vi "theOne_V2.vi"() -> ()   [LabVIEW 2021]
uses:
  <userlib>/er4commlib_labview/er4commlib_labview.lvlib
panel:
  in  "acqFlag":bool
  in  "purgeFlag":bool
  out "DataCh1":dbl[](graph)
  out "DataCh2":dbl[](graph)
  out "DataCh3":dbl[](graph)
  out "DataCh4":dbl[](graph)
  out "VolAndTrig":dbl[][](graph)
  out "triggerImage":picture
  in  "path to triggerImage file jpg":path=path "C:/neoDiag/MrAnderson/Img/trigger.jpg"
  in  "Trigger":T1={"manual start"=FALSE, "duration [us]"=200.0, "period [ms]"=1.0, "delay [us]"=0.0, "reps"=1000, "active"=TRUE} {"delay [us]" format="%_5f"; "period [ms]" format="%_5f"; "duration [us]" format="%_5f"}
  in  "Voltage Stimulus":T2={"stimulus"=FALSE, "Vhold [mV]"=-50.0, "Vpulse [mV]"=0.0, "Vstep [mV]"=10.0, "N"=10, "Thold [ms]"=0.0, "Tpulse [ms]"=200.0} {"Tpulse [ms]" format="%_5f"; "Thold [ms]" format="%_5f"; "Vstep [mV]" format="%_5f"; "Vpulse [mV]" format="%_5f"; "Vhold [mV]" format="%_5f"}
  in  "acquire data":bool
  in  "stop":bool
  out "pulseTrainImage":picture
  in  "path to pulseTrainImage file jpg":path=path "C:/neoDiag/MrAnderson/Img/volProtVarAmpl.jpg"
  in  "Tab Control":enum32{"AcqPara", "AdvPara"}(tab)
  in  "Acquisition Parameters":T3={"Camera "=FALSE, "Period [ms]"=200.0, "Duration [ms]"=0.2, "Delay [ms]"=0.0, "Pulses [#]"=10, "sampling rate [kHz]"="1,25", "current range [nA]"="2", "time [s]"=2.0} {"Delay [ms]" format="%_5f"; "Duration [ms]" format="%_5f"; "Period [ms]" format="%_5f"}
  in  "advancedSettings":T4={"Channels to read"=6, "update rate of read data loop"=100, "displayRange"=512}
  out "Error Out Int":u32
  out "Error Out String":string="clean"
  out "E4 parameters":T5={"currentChannelsNum out"=1, "voltageChannelsNum out"=4, "gpChannelsNum out"=1, "sampling rate [kHz]"=1.25, "real sampling rate [kHz]"=1.220703125, "Ch_min"=-2.0, "Ch_max"=2.0, "Ch_step"=6.103701895199438e-05, "Ch_unit"=1e-09}
  in  "Display 1":cluster{"ChArray":bool[]}={"ChArray"=[FALSE, TRUE, TRUE, TRUE, FALSE, FALSE]}
  out "Error Read":errorcluster
  # "DataCh1"
  # "DataCh2"
  # "DataCh3"
  # "DataCh4"
  # "Voltage"
  # "Trigger"
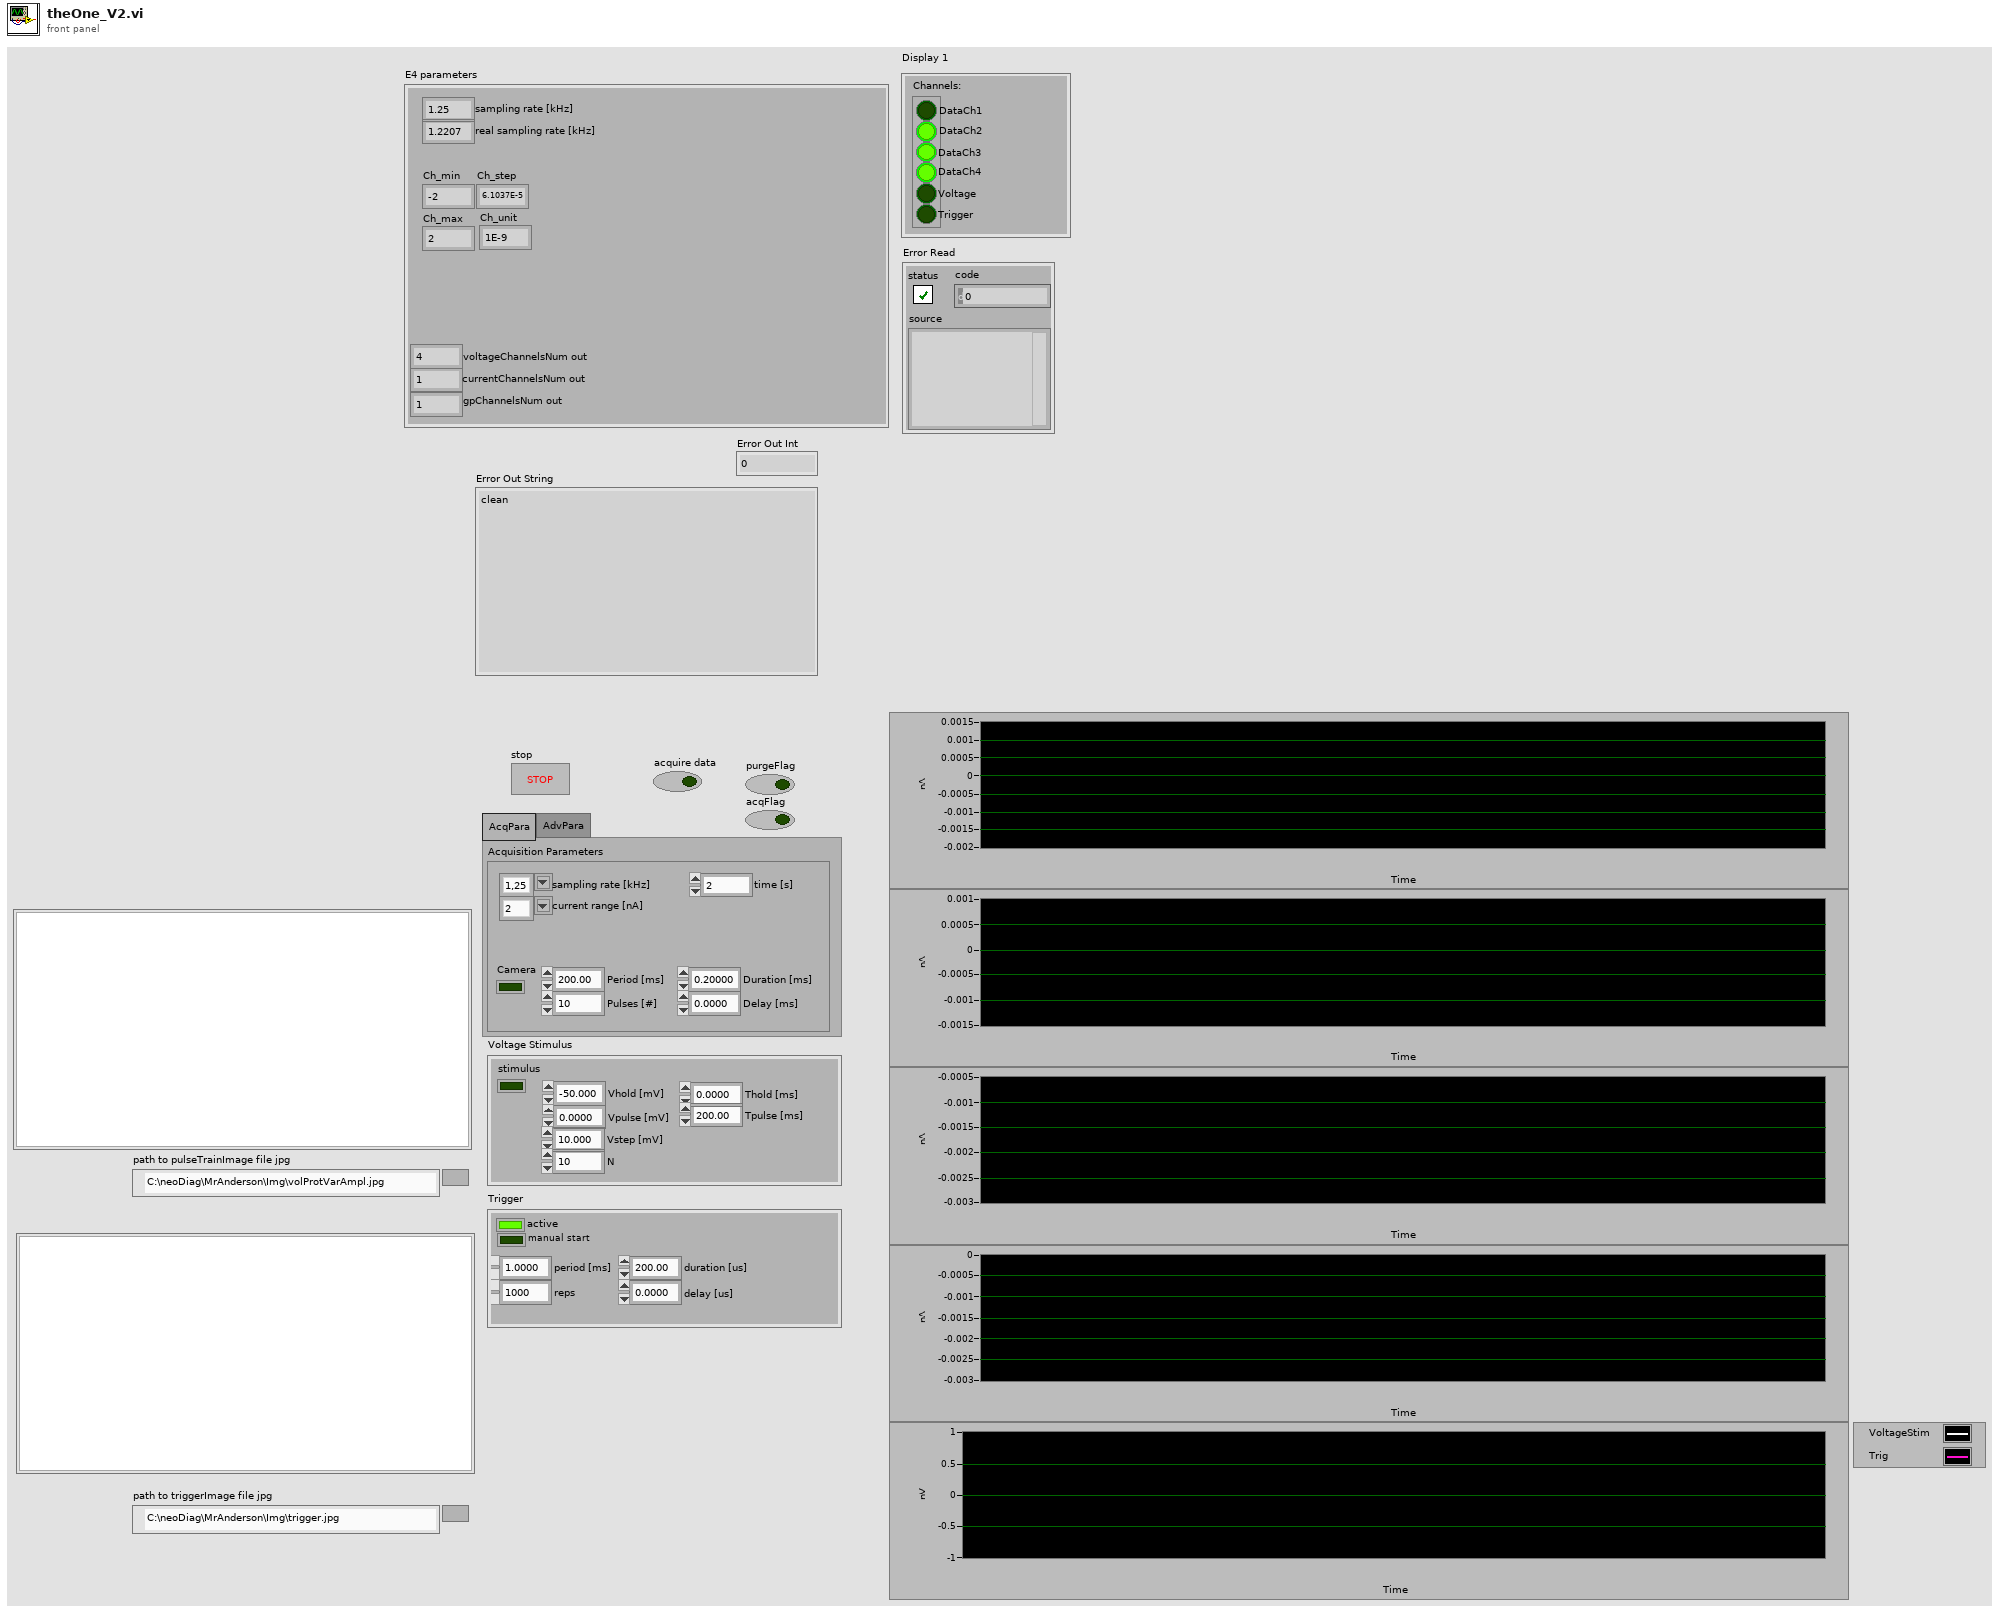
[diagram p1: front panel]
types:
  T1 = cluster{"manual start":bool, "duration [us]":dbl, "period [ms]":dbl, "delay [us]":dbl, "reps":u32, "active":bool}
  T2 = cluster{"stimulus":bool, "Vhold [mV]":dbl, "Vpulse [mV]":dbl, "Vstep [mV]":dbl, "N":u32, "Thold [ms]":dbl, "Tpulse [ms]":dbl}
  T3 = cluster{"Camera ":bool, "Period [ms]":dbl, "Duration [ms]":dbl, "Delay [ms]":dbl, "Pulses [#]":u32, "sampling rate [kHz]":string, "current range [nA]":string, "time [s]":dbl}
  T4 = cluster{"Channels to read":i32, "update rate of read data loop":i32, "displayRange":i32}
  T5 = cluster{"currentChannelsNum out":u32, "voltageChannelsNum out":u32, "gpChannelsNum out":u32, "sampling rate [kHz]":dbl, "real sampling rate [kHz]":dbl, "Ch_min":dbl, "Ch_max":dbl, "Ch_step":dbl, "Ch_unit":dbl}
  T6 = typedef "imagedata.ctl" = cluster{"image type":i32, "image depth":i32, "image":u8[], "mask":u8[], "colors":u32[], "Rectangle":cluster{"left":i16, "top":i16, "right":i16, "bottom":i16}}
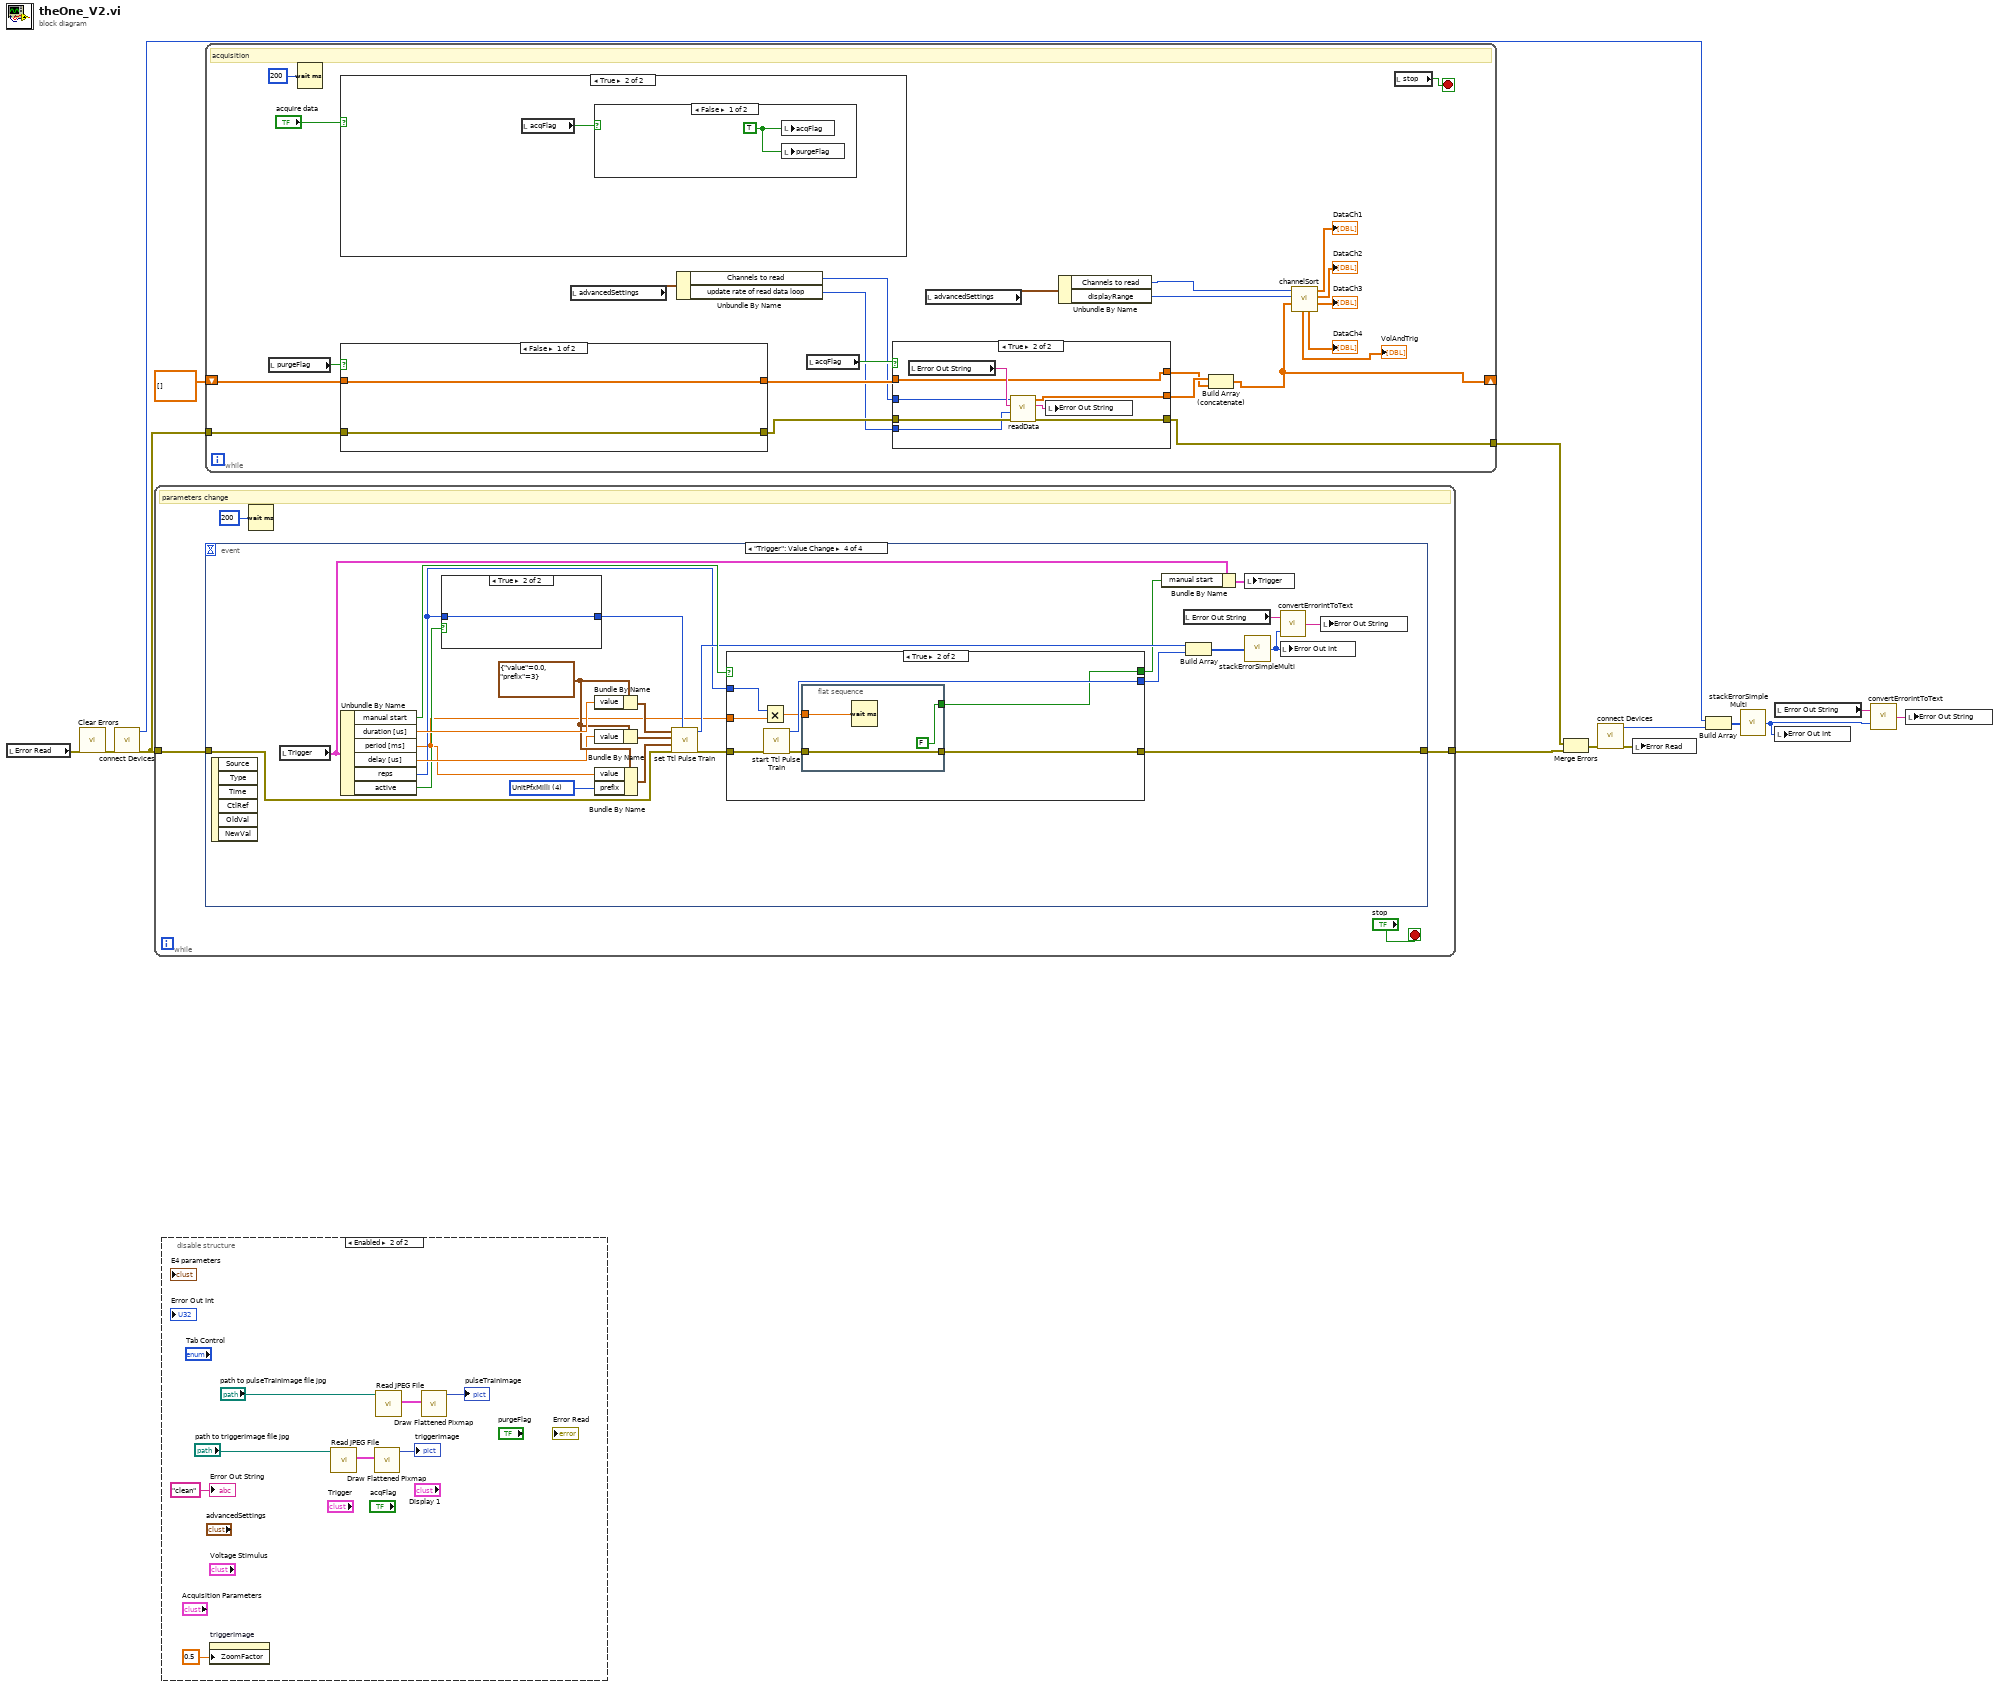
[diagram p0: block diagram]
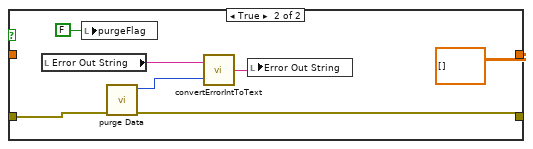
[diagram p2: hidden frame]
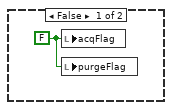
[diagram p3: hidden frame]
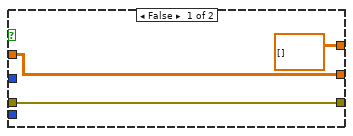
[diagram p5: hidden frame]
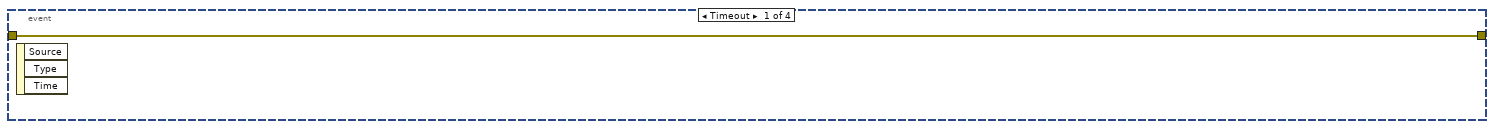
[diagram p6: hidden frame]
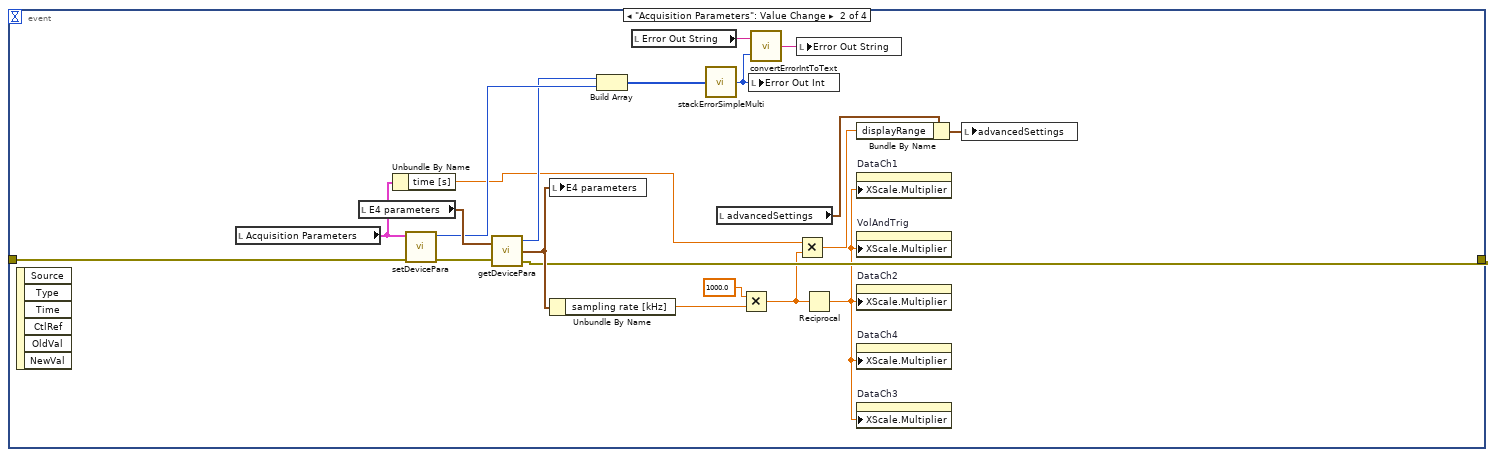
[diagram p7: hidden frame]
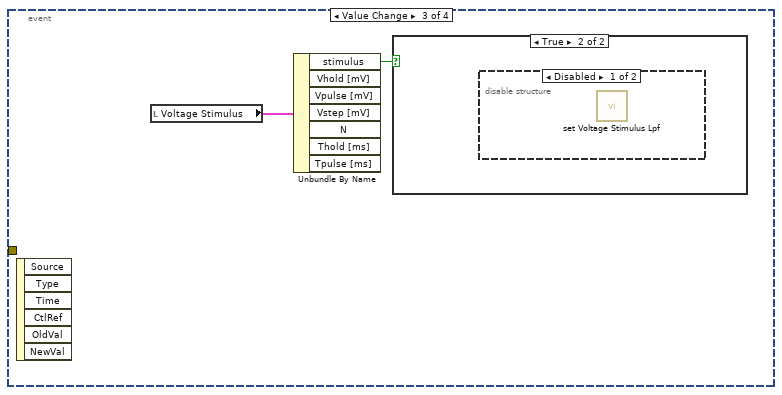
[diagram p8: hidden frame]
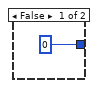
[diagram p11: hidden frame]
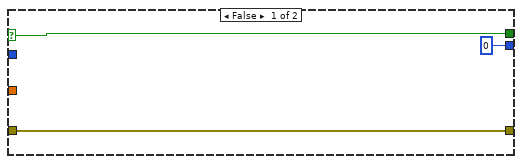
[diagram p12: hidden frame]
diagram:
  n1 = local read "Error Read"() -> (w13:errorcluster)
  n2 = call <vilib>:"Clear Errors.vi"("error in (no error)"=w13) -> ("error out"=w11:errorcluster)  [unwired: 5 in, 1 out]
  n3 = call <userlib>:"connect Devices.vi"("error in (no error)"=w11) -> ("error out"=w2:errorcluster, "function return"=w3:u32)  [unwired: 9 in]
  n4 = while {
    tunnel: w2 -> [w16]
    tunnel: [w15] -> w1
    stop <- "stop" stop-if-true
    # "parameters change"
    n5 = event shown="[3] \"Trigger\": Value Change" {
      selector: _ -> [_ _ _ _]
      dyn-events: _ -> [_ _ _ _]
      timeout: _ -> [_ _ _ _]
      tunnel: [w19 w32 _ w64] -> w15
      tunnel: w16 -> [w19 w31 _ w56]
      event Timeout {
        n6 = event-data() -> ()  [unwired: 1 in, 3 out]
      }
      event "Acquisition Parameters": Value Change {
        n7 = event-data() -> ()  [unwired: 1 in, 6 out]
        n8 = local read "Acquisition Parameters"() -> (w25:T3)
        n9 = local read "E4 parameters"() -> (w34:T5)
        n10 = Unbundle By Name(w25) -> ("time [s]"=w24:dbl)
        n11 = call "setDevicePara.vi"("error in (no error)"=w31, "Acquisition Parameters 2"=w25) -> ("error out"=w38:errorcluster, "function return"=w30:u32)  [unwired: 8 in]
        n12 = call "getDevicePara.vi"("Seetings in"=w34, "error in (no error)"=w38) -> ("Error Out"=w29:u32, "Seetings out"=w37:T5, "error out"=w32:errorcluster)
        n13 = local write "E4 parameters"(w37) -> ()
        n14 = Unbundle By Name(w37) -> ("sampling rate [kHz]"=w39:dbl)
        n15 = Build Array(w29, w30) -> (w28:u32[])
        n16 = local read "Error Out String"() -> (w36:string)
        n17 = call "stackErrorSimpleMulti.vi"("Error List"=w28) -> ("Error Out"=w27:u32)
        n18 = local read "advancedSettings"() -> (w20:T4)
        n19 = Multiply(x=1000.0, y=w39) -> (x*y=w23:dbl)
        n20 = local write "Error Out Int"(w27) -> ()
        n21 = call "convertErrorIntToText.vi"("Error Int In (function return)"=w27, "Error String In"=w36) -> ("Error String Out"=w35:string)
        n22 = local write "Error Out String"(w35) -> ()
        n23 = Multiply(x=w24, y=w23) -> (x*y=w21:dbl)
        n24 = Reciprocal(x=w23) -> (1/x=w26:dbl)
        n25 = Bundle By Name(cluster=w20, "displayRange"=w21) -> (w22:T4)
        n26 = property on="DataCh1" class="WFGraph (strict)"("XScale.Multiplier"=w26) -> ()  [unwired: 2 in, 2 out]
        n27 = property on="VolAndTrig" class="WFGraph (strict)"("XScale.Multiplier"=w26) -> ()  [unwired: 2 in, 2 out]
        n28 = property on="DataCh2" class="WFGraph (strict)"("XScale.Multiplier"=w26) -> ()  [unwired: 2 in, 2 out]
        n29 = property on="DataCh4" class="WFGraph (strict)"("XScale.Multiplier"=w26) -> ()  [unwired: 2 in, 2 out]
        n30 = property on="DataCh3" class="WFGraph (strict)"("XScale.Multiplier"=w26) -> ()  [unwired: 2 in, 2 out]
        n31 = local write "advancedSettings"(w22) -> ()
      }
      event "Voltage Stimulus.stimulus": Value Change {
        n32 = event-data() -> ()  [unwired: 1 in, 6 out]
        n33 = local read "Voltage Stimulus"() -> (w41:T2)
        n34 = Unbundle By Name(w41) -> ("stimulus"=w40:bool)  [unwired: 6 out]
        n35 = case shown="True" w40 {
          frame False {
          }
          frame True {
            n36 = disable-structure shown="Disabled" {
              frame Disabled {
                n37 = call <userlib>:"set Voltage Stimulus Lpf.vi"() -> ()  [unwired: 10 in, 2 out]
              }
              frame Enabled {
              }
            }
          }
        }
      }
      event "Trigger": Value Change {
        w59 = cluster{"value":dbl, "prefix":u32} {"value"=0.0, "prefix"=3} ("pulseDuration")
        w63 = u32 4 items=["UnitPfxFemto", "UnitPfxPico", "UnitPfxNano", "UnitPfxMicro", "UnitPfxMilli", "UnitPfxNone", "UnitPfxKilo", "UnitPfxMega", "UnitPfxGiga", "UnitPfxTera", "UnitPfxPeta", "UnitPfxNum"] ("prefix")
        n38 = event-data() -> ()  [unwired: 1 in, 6 out]
        n39 = local read "Trigger"() -> (w46:T1)
        n40 = Unbundle By Name(w46) -> ("manual start"=w65:bool, "duration [us]"=w61:dbl, "period [ms]"=w42:dbl, "delay [us]"=w58:dbl, "reps"=w43:u32, "active"=w54:bool)
        n41 = case shown="True" w54 {
          tunnel: w43 -> [_ w67]
          tunnel: [u32 0 ("reps") w67] -> w53
          frame False {
          }
          frame True {
          }
        }
        n42 = Bundle By Name(cluster=w59, "value"=w61) -> (w60:cluster{"value":dbl, "prefix":u32})
        n43 = Bundle By Name(cluster=w59, "value"=w58) -> (w57:cluster{"value":dbl, "prefix":u32})
        n44 = Bundle By Name(cluster=w59, "value"=w42, "prefix"=w63) -> (w62:cluster{"value":dbl, "prefix":u32})
        n45 = call <userlib>:"set Ttl Pulse Train.vi"("numberOfPulses"=w53, "error in (no error)"=w56, "period"=w62, "pulseDelay"=w57, "pulseDuration"=w60) -> ("error out"=w55:errorcluster, "function return"=w49:u32)  [unwired: 5 in]
        n46 = case shown="True" w65 {
          selector: w65 -> [w68 _]
          tunnel: w55 -> [w70 w78]
          tunnel: [w70 w74] -> w64
          tunnel: [u32 0 ("function return") w77] -> w48
          tunnel: [w68 w76] -> w45
          tunnel: w43 -> [_ w73]
          tunnel: w42 -> [_ w72]
          frame False {
          }
          frame True {
            n47 = Multiply(x=w73, y=w72) -> (x*y=w71:dbl)
            n48 = call <userlib>:"start Ttl Pulse Train.vi"("error in (no error)"=w78) -> ("error out"=w75:errorcluster, "function return"=w77:u32)  [unwired: 9 in]
            n49 = flat-sequence {
              tunnel: [FALSE] -> w76
              tunnel: w75 -> [w80]
              tunnel: [w80] -> w74
              tunnel: w71 -> [w79]
              frame #0 {
                n50 = Wait (ms)(milliseconds to wait=w79) -> ()  [unwired: 1 out]
              }
            }
          }
        }
        n51 = Bundle By Name(cluster=w46, "manual start"=w45) -> (w44:T1)
        n52 = local read "Error Out String"() -> (w47:string)
        n53 = Build Array(w49, w48) -> (w51:u32[])
        n54 = local write "Trigger"(w44) -> ()
        n55 = call "stackErrorSimpleMulti.vi"("Error List"=w51) -> ("Error Out"=w50:u32)
        n56 = call "convertErrorIntToText.vi"("Error Int In (function return)"=w50, "Error String In"=w47) -> ("Error String Out"=w52:string)
        n57 = local write "Error Out Int"(w50) -> ()
        n58 = local write "Error Out String"(w52) -> ()
      }
    }
    n59 = Wait (ms)(milliseconds to wait=u32 200) -> ()  [unwired: 1 out]
  }
  n60 = disable-structure shown="Enabled" {
    frame Disabled {
    }
    frame Enabled {
      n61 = property on="triggerImage" class="Pict"("ZoomFactor"=sgl 0.5 ("Zoom Factor")) -> ()  [unwired: 2 in, 2 out]
      n62 = call <vilib>:"Read JPEG File.vi"("path to JPEG file"="path to triggerImage file jpg") -> ("image data"=w85:T6)  [unwired: 8 in, 2 out]
      n63 = call <vilib>:"Draw Flattened Pixmap.vi"("image data"=w85) -> ("new picture"=→"triggerImage":picture)  [unwired: 8 in]
      n64 = call <vilib>:"Read JPEG File.vi"("path to JPEG file"="path to pulseTrainImage file jpg") -> ("image data"=w88:T6)  [unwired: 8 in, 2 out]
      n65 = call <vilib>:"Draw Flattened Pixmap.vi"("image data"=w88) -> ("new picture"=→"pulseTrainImage":picture)  [unwired: 8 in]
      "Error Out String" <- "clean" ("Error String Out")
    }
  }
  n66 = while {
    tunnel: w2 -> [w106]
    shift-right: [w90] -> _
    shift-left: dbl[][] [] -> [w105]
    tunnel: [w102] -> w12
    stop <- w110 stop-if-true
    # "acquisition"
    n67 = local read "purgeFlag"() -> (w108:bool)
    n68 = Wait (ms)(milliseconds to wait=u32 200) -> ()  [unwired: 1 out]
    n69 = case shown="True" "acquire data" {
      frame False {
        w123 = FALSE
        n70 = local write "acqFlag"(w123) -> ()
        n71 = local write "purgeFlag"(w123) -> ()
      }
      frame True {
        n72 = local read "acqFlag"() -> (w124:bool)
        n73 = case shown="False" w124 {
          frame False {
            w125 = TRUE
            n74 = local write "acqFlag"(w125) -> ()
            n75 = local write "purgeFlag"(w125) -> ()
          }
          frame True {
          }
        }
      }
    }
    n76 = case shown="False" w108 {
      tunnel: w106 -> [w115 w119]
      tunnel: [w115 w118] -> w103
      tunnel: [w114 dbl[][] [] ("Array")] -> w104
      tunnel: w105 -> [w114 _]
      frame False {
      }
      frame True {
        n77 = local read "Error Out String"() -> (w122:string)
        n78 = local write "purgeFlag"(FALSE) -> ()
        n79 = call <userlib>:"purge Data.vi"("error in (no error)"=w119) -> ("error out"=w118:errorcluster, "function return"=w120:u32)  [unwired: 9 in]
        n80 = call "convertErrorIntToText.vi"("Error Int In (function return)"=w120, "Error String In"=w122) -> ("Error String Out"=w121:string)
        n81 = local write "Error Out String"(w121) -> ()
      }
    }
    n82 = local read "advancedSettings"() -> (w101:T4)
    n83 = Unbundle By Name(w101) -> ("Channels to read"=w100:i32, "update rate of read data loop"=w99:i32)
    n84 = local read "acqFlag"() -> (w109:bool)
    n85 = case shown="True" w109 {
      tunnel: w103 -> [w126 w136]
      tunnel: [w128 w135] -> w112
      tunnel: w100 -> [_ w132]
      tunnel: w99 -> [_ w131]
      tunnel: w104 -> [w128 w130]
      tunnel: [dbl[][] [] ("Array") w130] -> w111
      tunnel: [w126 w129] -> w102
      frame False {
      }
      frame True {
        n86 = local read "Error Out String"() -> (w134:string)
        n87 = call "readData.vi"("error in (no error)"=w136, "time readout loops [ms]"=w131, "Error String Out in"=w134, "Channels"=w132) -> ("error out"=w129:errorcluster, "Error String Out out"=w133:string, "Array"=w135:dbl[][])  [unwired: 5 in]
        n88 = local write "Error Out String"(w133) -> ()
      }
    }
    n89 = local read "advancedSettings"() -> (w93:T4)
    n90 = Unbundle By Name(w93) -> ("Channels to read"=w92:i32, "displayRange"=w91:i32)
    n91 = Build Array (concatenate)(w112, w111) -> (w90:dbl[][])
    n92 = call "channelSort.vi"("Array 7"=w90, "displayRange"=w91, "Channels to read"=w92) -> ("Array 4"=→"DataCh3":dbl[], "Array 3"=→"DataCh2":dbl[], "Array 2"=→"DataCh1":dbl[], "Array 5"=→"DataCh4":dbl[], "Array 6"=→"VolAndTrig":dbl[][])  [unwired: 3 in, 1 out]
    n93 = local read "stop"() -> (w110:bool)
  }
  n94 = Merge Errors(w12, w1) -> (w10:errorcluster)
  n95 = call <userlib>:"connect Devices.vi"("error in (no error)"=w10) -> ("error out"=w9:errorcluster, "function return"=w5:u32)  [unwired: 9 in]
  n96 = local write "Error Read"(w9) -> ()
  n97 = Build Array(w3, w5) -> (w7:u32[])
  n98 = call "stackErrorSimpleMulti.vi"("Error List"=w7) -> ("Error Out"=w8:u32)
  n99 = local read "Error Out String"() -> (w4:string)
  n100 = local write "Error Out Int"(w8) -> ()
  n101 = call "convertErrorIntToText.vi"("Error Int In (function return)"=w8, "Error String In"=w4) -> ("Error String Out"=w6:string)
  n102 = local write "Error Out String"(w6) -> ()
